vi "Digital Input Data.vi"(8 "error in (no error)":errorcluster, 10 "Digital Data":bool[](array[boolean]), 11 "Digital Input Data in":refnum<class "Digital Input Data.lvclass">) -> (0 "error out":errorcluster, 3 "Digital Input Data out":refnum<class "Digital Input Data.lvclass">)   [LabVIEW 2024, in "DAQmx Actor Interface.lvlib" / "Digital Input Data.lvclass"]
uses:
  Digital Input Data.lvclass
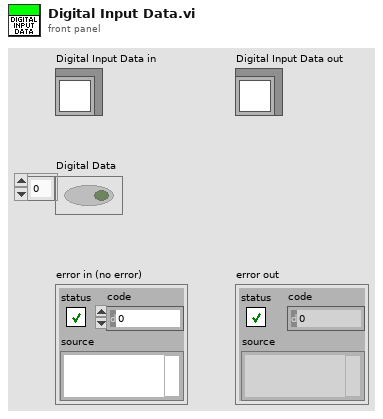
[diagram p1: front panel]
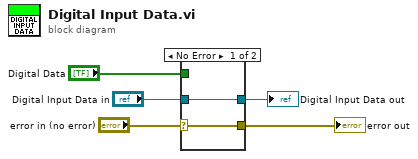
[diagram p0: block diagram]
diagram:
  n1 = case shown="No Error" "error in (no error)" {
    selector: "error in (no error)" -> [w6 w9]
    tunnel: [w6 w9] -> w4
    tunnel: [w7 w8] -> w2
    tunnel: "Digital Input Data in" -> [w7 w8]
    tunnel: "Digital Data" -> [_ _]
    frame No Error {
    }
    frame Error {
    }
  }
  "error out" <- w4
  "Digital Input Data out" <- w2
